vi "Calculate Terminals Needed.vi"(11 "Instrument Driver Method Descriptor Array":T1) -> (2 "No. Outputs":i32, 3 "No. Inputs":i32)   [LabVIEW 2021]
uses:
  <vilib>/myRIO/Common/Express VI Framework/typedefs/Instrument Driver Method Descriptor Array.ctl
  <vilib>/myRIO/Common/Express VI Framework/typedefs/Instrument Driver Method Descriptor.ctl
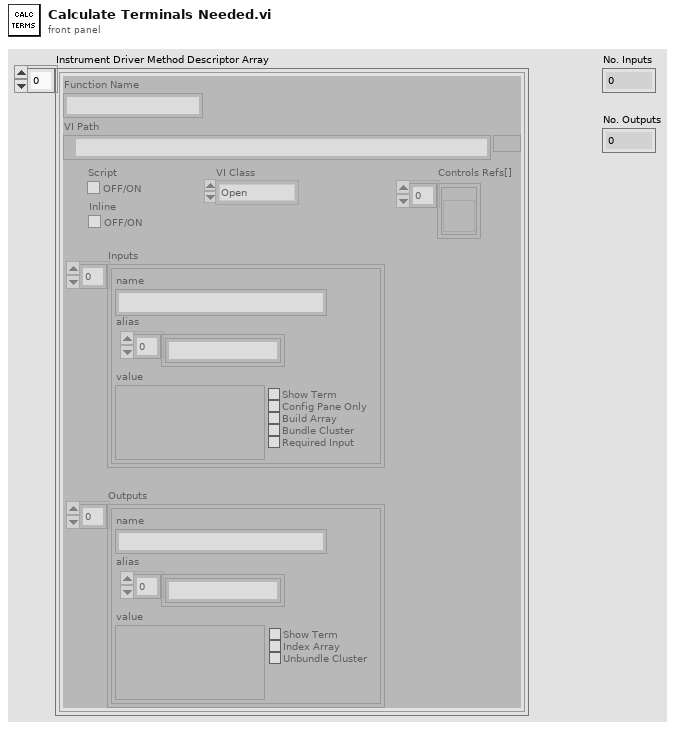
[diagram p1: front panel]
types:
  T1 = typedef "Instrument Driver Method Descriptor Array.ctl" = T2[]
  T2 = typedef "Instrument Driver Method Descriptor.ctl" = cluster{"Function Name":string, "VI Path":path, "Script":bool, "Inputs":cluster{"name":string, "value":variant, "Config Pane Only":bool, "Build Array":bool, "Bundle Cluster":bool, "Show Term":bool, "alias":string[], "Required Input":bool}[], "Outputs":cluster{"name":string, "value":variant, "Show Term":bool, "Index Array":bool, "Unbundle Cluster":bool, "alias":string[]}[], "VI Class":enum16{"Open", "Configure", "Data", "Manage", "Close"}, "Controls Refs[]":refnum<vi>[], "Inline":bool}
  T3 = cluster{"name":string, "value":variant, "Show Term":bool, "Index Array":bool, "Unbundle Cluster":bool, "alias":string[]}[]
  T4 = cluster{"name":string, "value":variant, "Config Pane Only":bool, "Build Array":bool, "Bundle Cluster":bool, "Show Term":bool, "alias":string[], "Required Input":bool}[]
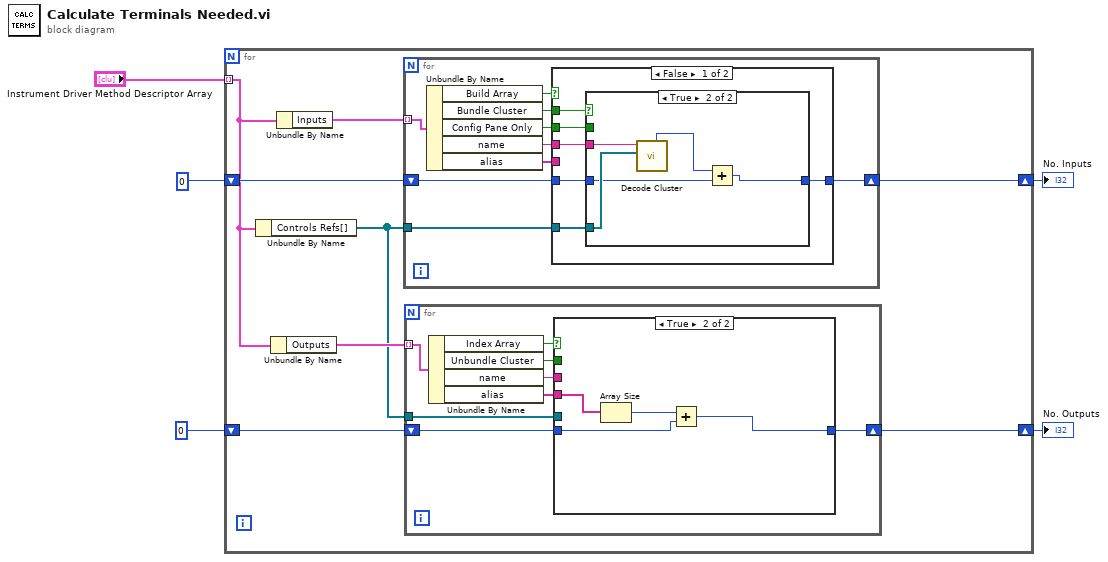
[diagram p0: block diagram]
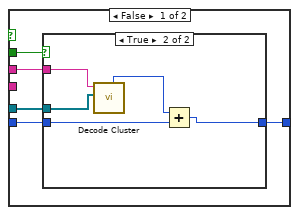
[diagram p2: hidden frame]
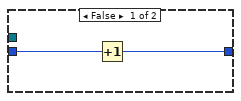
[diagram p3: hidden frame]
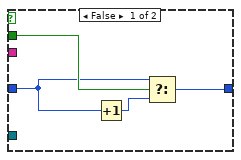
[diagram p4: hidden frame]
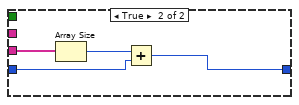
[diagram p5: hidden frame]
diagram:
  n1 = for {
    tunnel: "Instrument Driver Method Descriptor Array" -> [w9] mode=indexing
    shift-right: [w10] -> w2
    shift-left: 0 -> [w11]
    shift-right: [w7] -> w1
    shift-left: 0 -> [w8]
    n2 = Unbundle By Name(w9) -> ("Controls Refs[]"=w6:refnum<vi>[])
    n3 = Unbundle By Name(w9) -> ("Outputs"=w13:T3)
    n4 = Unbundle By Name(w9) -> ("Inputs"=w12:T4)
    n5 = for {
      tunnel: w12 -> [w46] mode=indexing
      shift-right: [w41] -> w10
      shift-left: w11 -> [w42]
      tunnel: w6 -> [w38]
      n6 = Unbundle By Name(w46) -> ("Build Array"=w45:bool, "Bundle Cluster"=w40:bool, "Config Pane Only"=w39:bool, "name"=w44:string, "alias"=w43:string[])
      n7 = case shown="False" w45 {
        tunnel: w44 -> [w50 _]
        tunnel: w43 -> [_ w65]
        tunnel: w42 -> [w48 w63]
        tunnel: [w47 w62] -> w41
        tunnel: w40 -> [w52 _]
        tunnel: w39 -> [w51 _]
        tunnel: w38 -> [w49 _]
        frame False {
          n8 = case shown="True" w52 {
            tunnel: w51 -> [w56 _]
            tunnel: w50 -> [_ w61]
            tunnel: w49 -> [_ w60]
            tunnel: w48 -> [w55 w59]
            tunnel: [w53 w58] -> w47
            frame False {
              n9 = Increment(x=w55) -> (x+1=w54:i32)
              n10 = Select(t=w55, s=w56, f=w54) -> (s? t:f=w53:i32)
            }
            frame True {
              n11 = call <vilib>:"Decode Cluster.vi"("Controls Refs[]"=w60, "Cluster Name"=w61) -> ("Cluster Size"=w57:i32)  [unwired: 5 in, 4 out]
              n12 = Add(x=w57, y=w59) -> (x+y=w58:i32)
            }
          }
        }
        frame True {
          n13 = Array Size(array=w65) -> (size(s)=w64:i32)
          n14 = Add(x=w64, y=w63) -> (x+y=w62:i32)
        }
      }
    }
    n15 = for {
      tunnel: w13 -> [w19] mode=indexing
      shift-right: [w16] -> w7
      shift-left: w8 -> [w17]
      tunnel: w6 -> [w14]
      n16 = Unbundle By Name(w19) -> ("Index Array"=w20:bool, "Unbundle Cluster"=w21:bool, "name"=w15:string, "alias"=w18:string[])
      n17 = case shown="True" w20 {
        tunnel: [w25 w36] -> w16
        tunnel: w21 -> [w26 _]
        tunnel: w18 -> [_ w35]
        tunnel: w17 -> [w22 w34]
        tunnel: w15 -> [w24 _]
        tunnel: w14 -> [w23 _]
        frame False {
          n18 = case shown="True" w26 {
            tunnel: [w27 w33] -> w25
            tunnel: w24 -> [_ w32]
            tunnel: w23 -> [_ w31]
            tunnel: w22 -> [w28 w30]
            frame False {
              n19 = Increment(x=w28) -> (x+1=w27:i32)
            }
            frame True {
              n20 = call <vilib>:"Decode Cluster.vi"("Controls Refs[]"=w31, "Cluster Name"=w32) -> ("Cluster Size"=w29:i32)  [unwired: 5 in, 4 out]
              n21 = Add(x=w29, y=w30) -> (x+y=w33:i32)
            }
          }
        }
        frame True {
          n22 = Array Size(array=w35) -> (size(s)=w37:i32)
          n23 = Add(x=w37, y=w34) -> (x+y=w36:i32)
        }
      }
    }
  }
  "No. Inputs" <- w2
  "No. Outputs" <- w1
